vi "Dashboard Main.vi"() -> ()   [LabVIEW 2023]
uses:
  <vilib>/event_ctls.llb/eventvkey.ctl
  <vilib>/Rock Robotics/WPI/ThirdParty/JAS_Junk/TrajLib/TypeDef/TRANSLATION2D.ctl
  d5e2e769-f078-4149-bfe1-3f7844503895.vi
  <vilib>/Rock Robotics/WPI/ThirdParty/JAS_Junk/TrajLib/Conv_Radians_Deg.vi
  <vilib>/Rock Robotics/WPI/ThirdParty/JAS_Junk/TrajLib/Conv_Deg_Radians.vi
  <vilib>/Rock Robotics/WPI/ThirdParty/JAS_Junk/TrajLib/Translation2d_Create.vi
  <vilib>/Rock Robotics/WPI/ThirdParty/JAS_Junk/TrajLib/Rotation2d_CreateXY.vi
  <vilib>/Rock Robotics/WPI/ThirdParty/JAS_Junk/TrajLib/VI/Util_GetTime_U32.vi
  <vilib>/Rock Robotics/WPI/ThirdParty/JAS_Junk/TrajLib/Util_CalcDist.vi
  <vilib>/Rock Robotics/Network Tables/NT Read Numeric Array.vi
  <vilib>/Rock Robotics/WPI/ThirdParty/JAS_Junk/TrajLib/VI/Util_GetTime_U64.vi
  <vilib>/Rock Robotics/WPI/Dashboard/WPI_DashboardLogging Global.vi
  <vilib>/picture/picture.llb/Draw True-Color Pixmap.vi
  <vilib>/Rock Robotics/WPI/ThirdParty/JAS_Junk/TrajLib/Trajectory_Library.lvlib
  <vilib>/vision/NI_Vision_Development_Module.lvlib
  <vilib>/Utility/miscctls.llb/LVPointDoubleTypeDef.ctl
panel:
  in  "FF on?":bool=TRUE
  in  "Arm/ArmLength_Meters":dbl
  in  "Arm/Mass_Kg":dbl
  in  "PID gains":T1
  in  "FF params":T2={"Kg_Gravity_gain"=0.5, "phi_Equilibrium_phase_Deg"=0.0, "Ks"=0.03}
  in  "Arm/ArmAngle_Dmd_Deg":dbl
  out "ArmAngle_Deg":dbl
  out "ArmSpeed_RadPerSec":dbl
  in  "Camera Settings Right":T3={"Frame Rate"=30, "Compression"=30, "Size"=1, "DB Camera Config"=FALSE} {"Frame Rate" scale=1.0..30.0; "Compression" scale=100.0..-1.0; "Size" items=["640x480", "320x240", "160x120"]}
  in  "Camera Name Right":string(combo)="No Camera Selection"
  out "Camera Perf":string
  in  "Camera Settings":T3={"Frame Rate"=30, "Compression"=30, "Size"=1, "DB Camera Config"=FALSE} {"Frame Rate" scale=1.0..30.0; "Compression" scale=100.0..-1.0; "Size" items=["640x480", "320x240", "160x120"]}
  in  "TCP":refnum<k5>
  in  "Rec Mode":enum32{"Stop", "Record", "Playback"}(radio)
  out "Robot IP":string
  out "Image Message":string="Timeout in Camera Communications"
  in  "Dashboard Tab":T4(tab)
  in  "Select Auto":string(combo)="Select Autonomous ..."
  out "NT Connection":bool
  out "MotorChart R":cluster{"Numeric":dbl, "Numeric":dbl}(graph)
  out "MotorChart L":cluster{"Numeric":dbl, "Numeric":dbl}(graph)
  out "MotorSliders R":cluster{"MotorSlide1":dbl, "MotorSlide2":dbl} {"MotorSlide2" scale=-1.0..1.0 scale format="%#_2e"; "MotorSlide1" scale=-1.0..1.0 scale format="%#_2e"}
  out "MotorSliders L":cluster{"MotorSlide1":dbl, "MotorSlide2":dbl} {"MotorSlide2" scale=-1.0..1.0 scale format="%#_2e"; "MotorSlide1" scale=-1.0..1.0 scale format="%#_2e"}
  out "Gyro":dbl(knob) scale=0.0..360.0
  out "JS1 Z":dbl(slide) scale=-1.0..1.0 scale format="%#_2e"
  out "JS1 Graph":cluster{"X":dbl, "Y":dbl}[](graph)
  out "JS1 Buttons":T5
  out "JS2 Z":dbl(slide) scale=-1.0..1.0 scale format="%#_2e"
  out "JS2 Graph":cluster{"X":dbl, "Y":dbl}[](graph)
  out "JS2 Buttons":T5
  out "Mode":T6(ring)=enum."Auto Disabled"
  out "Right Camera Perf":cluster{"Bandwidth (Mbps)":dbl, "FPS":dbl}
  out "Camera Image Right":T7(plugin-control)
  in  "DB/String 9":string
  in  "DB/String 8":string
  in  "DB/String 7":string
  in  "DB/String 6":string
  in  "DB/String 5":string
  in  "DB/String 4":string
  in  "DB/String 3":string
  in  "DB/String 2":string
  in  "DB/String 1":string
  in  "DB/String 0":string
  in  "DB/Slider 0":dbl(slide) scale=0.0..5.0
  in  "DB/Slider 1":dbl(slide) scale=0.0..5.0
  in  "DB/Slider 2":dbl(slide) scale=0.0..5.0
  in  "DB/Slider 3":dbl(slide) scale=0.0..5.0
  out "DB/LED 3":bool
  out "DB/LED 2":bool
  out "DB/LED 1":bool
  out "DB/LED 0":bool
  in  "DB/Button 3":bool
  in  "DB/Button 2":bool
  in  "DB/Button 1":bool
  in  "DB/Button 0":bool caption="New Name"
  out "Arm Graph":cluster{dbl[], dbl[]}[](graph)
  out "time":dbl
  out "Field":cluster{dbl[], dbl[]}[](graph)
  out "Current Time":dbl
  in  "Test Slider":dbl(slide) scale=0.0..100.0 scale format="%#_3g"
  in  "On/Off":bool caption="Solenoid"
  in  "Test Name":u16(ring) items=["Select the test to run..."]
  in  "Test Tree":string(tree)
  in  "Motor":cluster{"Value":dbl, "Enable":bool} {"Value" scale=-1.0..1.0 scale format="%#_3g"}
  out "Progress":T8 {"Test Progress" scale=0.0..100.0}
  in  "Rev/Fwd":cluster{"Forward":bool, "Reverse":bool}
  in  "Test Ring":u16(ring) items=["Monochrome", "Color"]
  in  "CheckList":i32(listbox)
  out "Tree":string(tree)
  out "Camera Image":T7(plugin-control)
  out "Background":bool
  in  "Camera Name":string(combo)="No Camera Selection"
  # "Motor Type: Falcon 500"
  # "Gear Ratio: 11.652"
  # "HW"
  # "HW"
  # "Joysticks"
  # "Drive Motors"
  # "Front"
  # "Right"
  # "Left"
  # "Back"
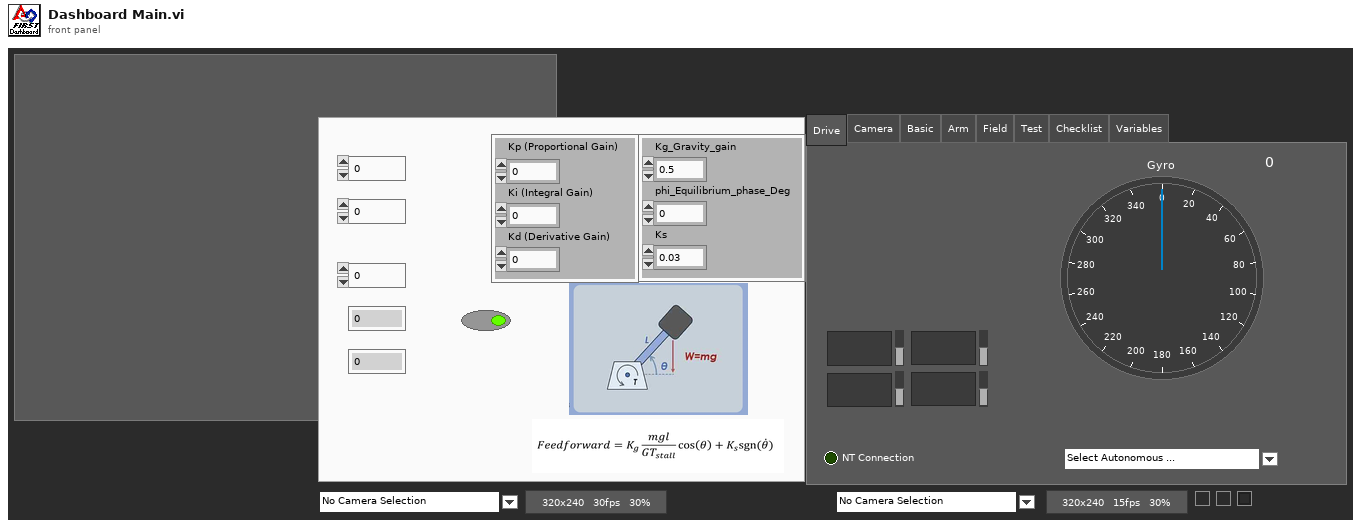
[diagram p1: front panel]
types:
  T1 = cluster{"Kp (Proportional Gain)":dbl, "Ki (Integral Gain)":dbl, "Kd (Derivative Gain)":dbl}
  T2 = cluster{"Kg_Gravity_gain":dbl, "phi_Equilibrium_phase_Deg":dbl, "Ks":dbl}
  T3 = cluster{"Frame Rate":i32, "Compression":i32, "Size":u16, "DB Camera Config":bool}
  T4 = enum32{"Drive", "Camera", "Basic", "Arm", "Field", "Test", "Checklist", "Variables"}
  T5 = cluster{bool, bool, bool, bool, bool, bool, bool, bool, bool, bool, bool, bool}
  T6 = enum8{"Tele-Op Disabled", "Tele-Op Enabled", "Auto Disabled", "Auto Enabled", "Test Disabled", "Test Enabled", "Disconnected", "No Code", "E-Stop"}
  T7 = typedef "IMAQ Image.ctl" = refnum<image>
  T8 = cluster{"Test Progress":u8, "Test Progress Text":string}
  T9 = typedef "Image Type" = u32
  T10 = cluster{"Save Path":path, "Interval (s)":dbl, "Keep":i32}
  T11 = enum32{"Drive", "Camera", "Basic", "Custom", "Test", "Commands", "Checklist", "Variables"}
  T12 = cluster{"Error Strings":string, "Disable Counts":cluster{u16, u16}, "Rail Faults":cluster{u16, u16, u16}, "Robot IP":string, "DB Mode":u8, "Event Info":cluster{"Name":string, "Type":u8, "Number":u16, "Replay":u8}}
  T13 = cluster{"Storage":cluster{"Disk Free":u64, "RAM Block":u32, "RAM free":u32}, "CPU Utilization":cluster{"CPU % ISR":sgl, "CPU % Time Crit":sgl, "CPU % Timed Str":sgl, "CPU % High":sgl, "CPU % Above":sgl, "CPU % Normal":sgl, "CPU % Low":sgl}, "CAN":cluster{"% Bus Utilization":sgl, "Bus Off Cnt":u32, "TX_FIFO Full Cnt":u32, "Receive Error Cnt":u8, "Transmit Error Cnt":u8}, "HID":cluster{"HID Outputs":u32, "Rumble Low":u16, "Rumble High":u16}[]}
  T14 = cluster{"Status bits":cluster{"Test Mode":bool, "Autonomous":bool, "Enabled":bool, "Code Start":bool, "Brownout":bool, "Reserved 2":bool, "Reserved 3":bool, "E-Stop":bool}, "Code Trace":cluster{"Disabled":bool, "TeleOp":bool, "Auto":bool, "Test":bool}, "Controller Type":enum16{"unknown", "cRIO", "roboRio"}, "Code?":enum16{"unknown", "noCode", "code"}, "Battery V":dbl}
  T15 = cluster{"Control Bits":cluster{"TestMode":bool, "Autonomous":bool, "Enabled":bool, "FMS Present":bool, bool, bool, bool, "E-Stop":bool}, "Team Station ":u8, "Countdown":sgl, "Joystick Values":cluster{"Axes":dbl[], "Buttons":bool[], "POVs":i16[]}[]}
  T16 = typedef "Trajectory_Library.lvlib/TRANSLATION2D.ctl" = cluster{"X":dbl, "Y":dbl}
  T17 = cluster{"Axes":dbl[], "Buttons":bool[], "POVs":i16[]}[]
  T18 = cluster{"Axes":dbl[], "Buttons":bool[], "POVs":i16[]}
  T19 = cluster{"Buttons[0]":bool, "Buttons[1]":bool, "Buttons[2]":bool, "Buttons[3]":bool, "Buttons[4]":bool, "Buttons[5]":bool, "Buttons[6]":bool, "Buttons[7]":bool, "Buttons[8]":bool, "Buttons[9]":bool, "Buttons[10]":bool, "Buttons[11]":bool}
  T20 = typedef "Trajectory_Library.lvlib/ROTATION2D.ctl" = cluster{"VALUE":dbl, "COS":dbl, "SIN":dbl}
  T21 = cluster{"Camera Image":refnum<vi>, "Dashboard Tab":refnum<vi>, "Background":refnum<vi>, "Rec Mode":refnum<vi>, "Test Slider":refnum<vi>, "On/Off ":refnum<vi>, "Test Ring":refnum<vi>, "Rev/Fwd":refnum<vi>, "Test Name":refnum<vi>, "Motor":refnum<vi>, "Progress":refnum<vi>, "CheckList":refnum<vi>, "Tree":refnum<vi>, "Test Tree":refnum<vi>, "Camera Settings":refnum<vi>, "Camera Name":refnum<vi>, "Camera Perf":refnum<vi>, "Camera Settings Right":refnum<vi>, "Camera Name Right":refnum<vi>, "Camera Image Right":refnum<vi>}
  T22 = cluster{"Global Rectangle":i32[], "Contours":cluster{"Contour Type":u32, "ROI Type":u32, "Points":i32[]}[]}
  T23 = cluster{"Camera Name":string, string, "Saved DB Images Info":cluster{"Save Path":path, "Interval (s)":dbl, "Keep":i32}}
  T24 = cluster{"Camera Name Right":string, string, "Saved DB Images Info":cluster{"Save Path":path, "Interval (s)":dbl, "Keep":i32}}
  T25 = cluster{"Operation":enum16{"Update", "Clear"}, "Color Box":u32}[]
  T26 = typedef "eventvkey.ctl" = enum16{"ASCII", "Enter", "Return", "Shift", "Ctrl", "Alt", "Cmd", "Opt", "Caps", "NumLock", "Clear", "Break", "Up", "Down", "Left", "Right", "Insert", "Delete", "Home", "End", "PageUp", "PageDown", "Escape", "Help", "Pause", "ScrollLock", "F1", "F2", "F3", "F4", "F5", "F6", "F7", "F8", "F9", "F10", "F11", "F12", "F13", "F14", "F15", "F16", "F17", "F18", "F19", "F20", "F21", "F22", "F23", "F24", "Play", "VolumeUp", "VolumeDown", "Mute", "Two Byte Char"}
  T27 = cluster{"Image Size":bool, "Image Type":bool, "Pixel Value":bool, "ROI Information":bool, "Zoom Factor":bool}
  T28 = cluster{"Operation":enum16{"Update", "Clear"}, "Color Box":u32}
  T29 = cluster{"Shift":bool, "Ctrl":bool, "Alt":bool, "Cmd":bool, "Opt":bool}
  T30 = typedef "imagedata.ctl" = cluster{"image type":i32, "image depth":i32, "image":u8[], "mask":u8[], "colors":u32[], "Rectangle":cluster{"left":i16, "top":i16, "right":i16, "bottom":i16}}
  T31 = typedef "LVPointDoubleTypeDef.ctl" = cluster{"X":dbl, "Y":dbl}
  T32 = typedef "LVCursorListTypeDef.ctl" = cluster{"Name":string, "Color":u32, "Style":u8, "Point Style":u8, "Name Visible":bool, "Allow Drag":bool, "Cursor Mode":u32, "Plot":i32, "Index":i32, "Position":cluster{"X":dbl, "Y":dbl}, "X Scale":u32, "Y Scale":u32, "Watch Plots":i32[], "Watch All Plots":bool, "Plot Area":i32, "Label Offset":cluster{"X":dbl, "Y":dbl}}[]
  T33 = cluster{"Name":string, "Color":u32, "Style":u8, "Point Style":u8, "Name Visible":bool, "Allow Drag":bool, "Cursor Mode":u32, "Plot":i32, "Index":i32, "Position":cluster{"X":dbl, "Y":dbl}, "X Scale":u32, "Y Scale":u32, "Watch Plots":i32[], "Watch All Plots":bool, "Plot Area":i32, "Label Offset":cluster{"X":dbl, "Y":dbl}}
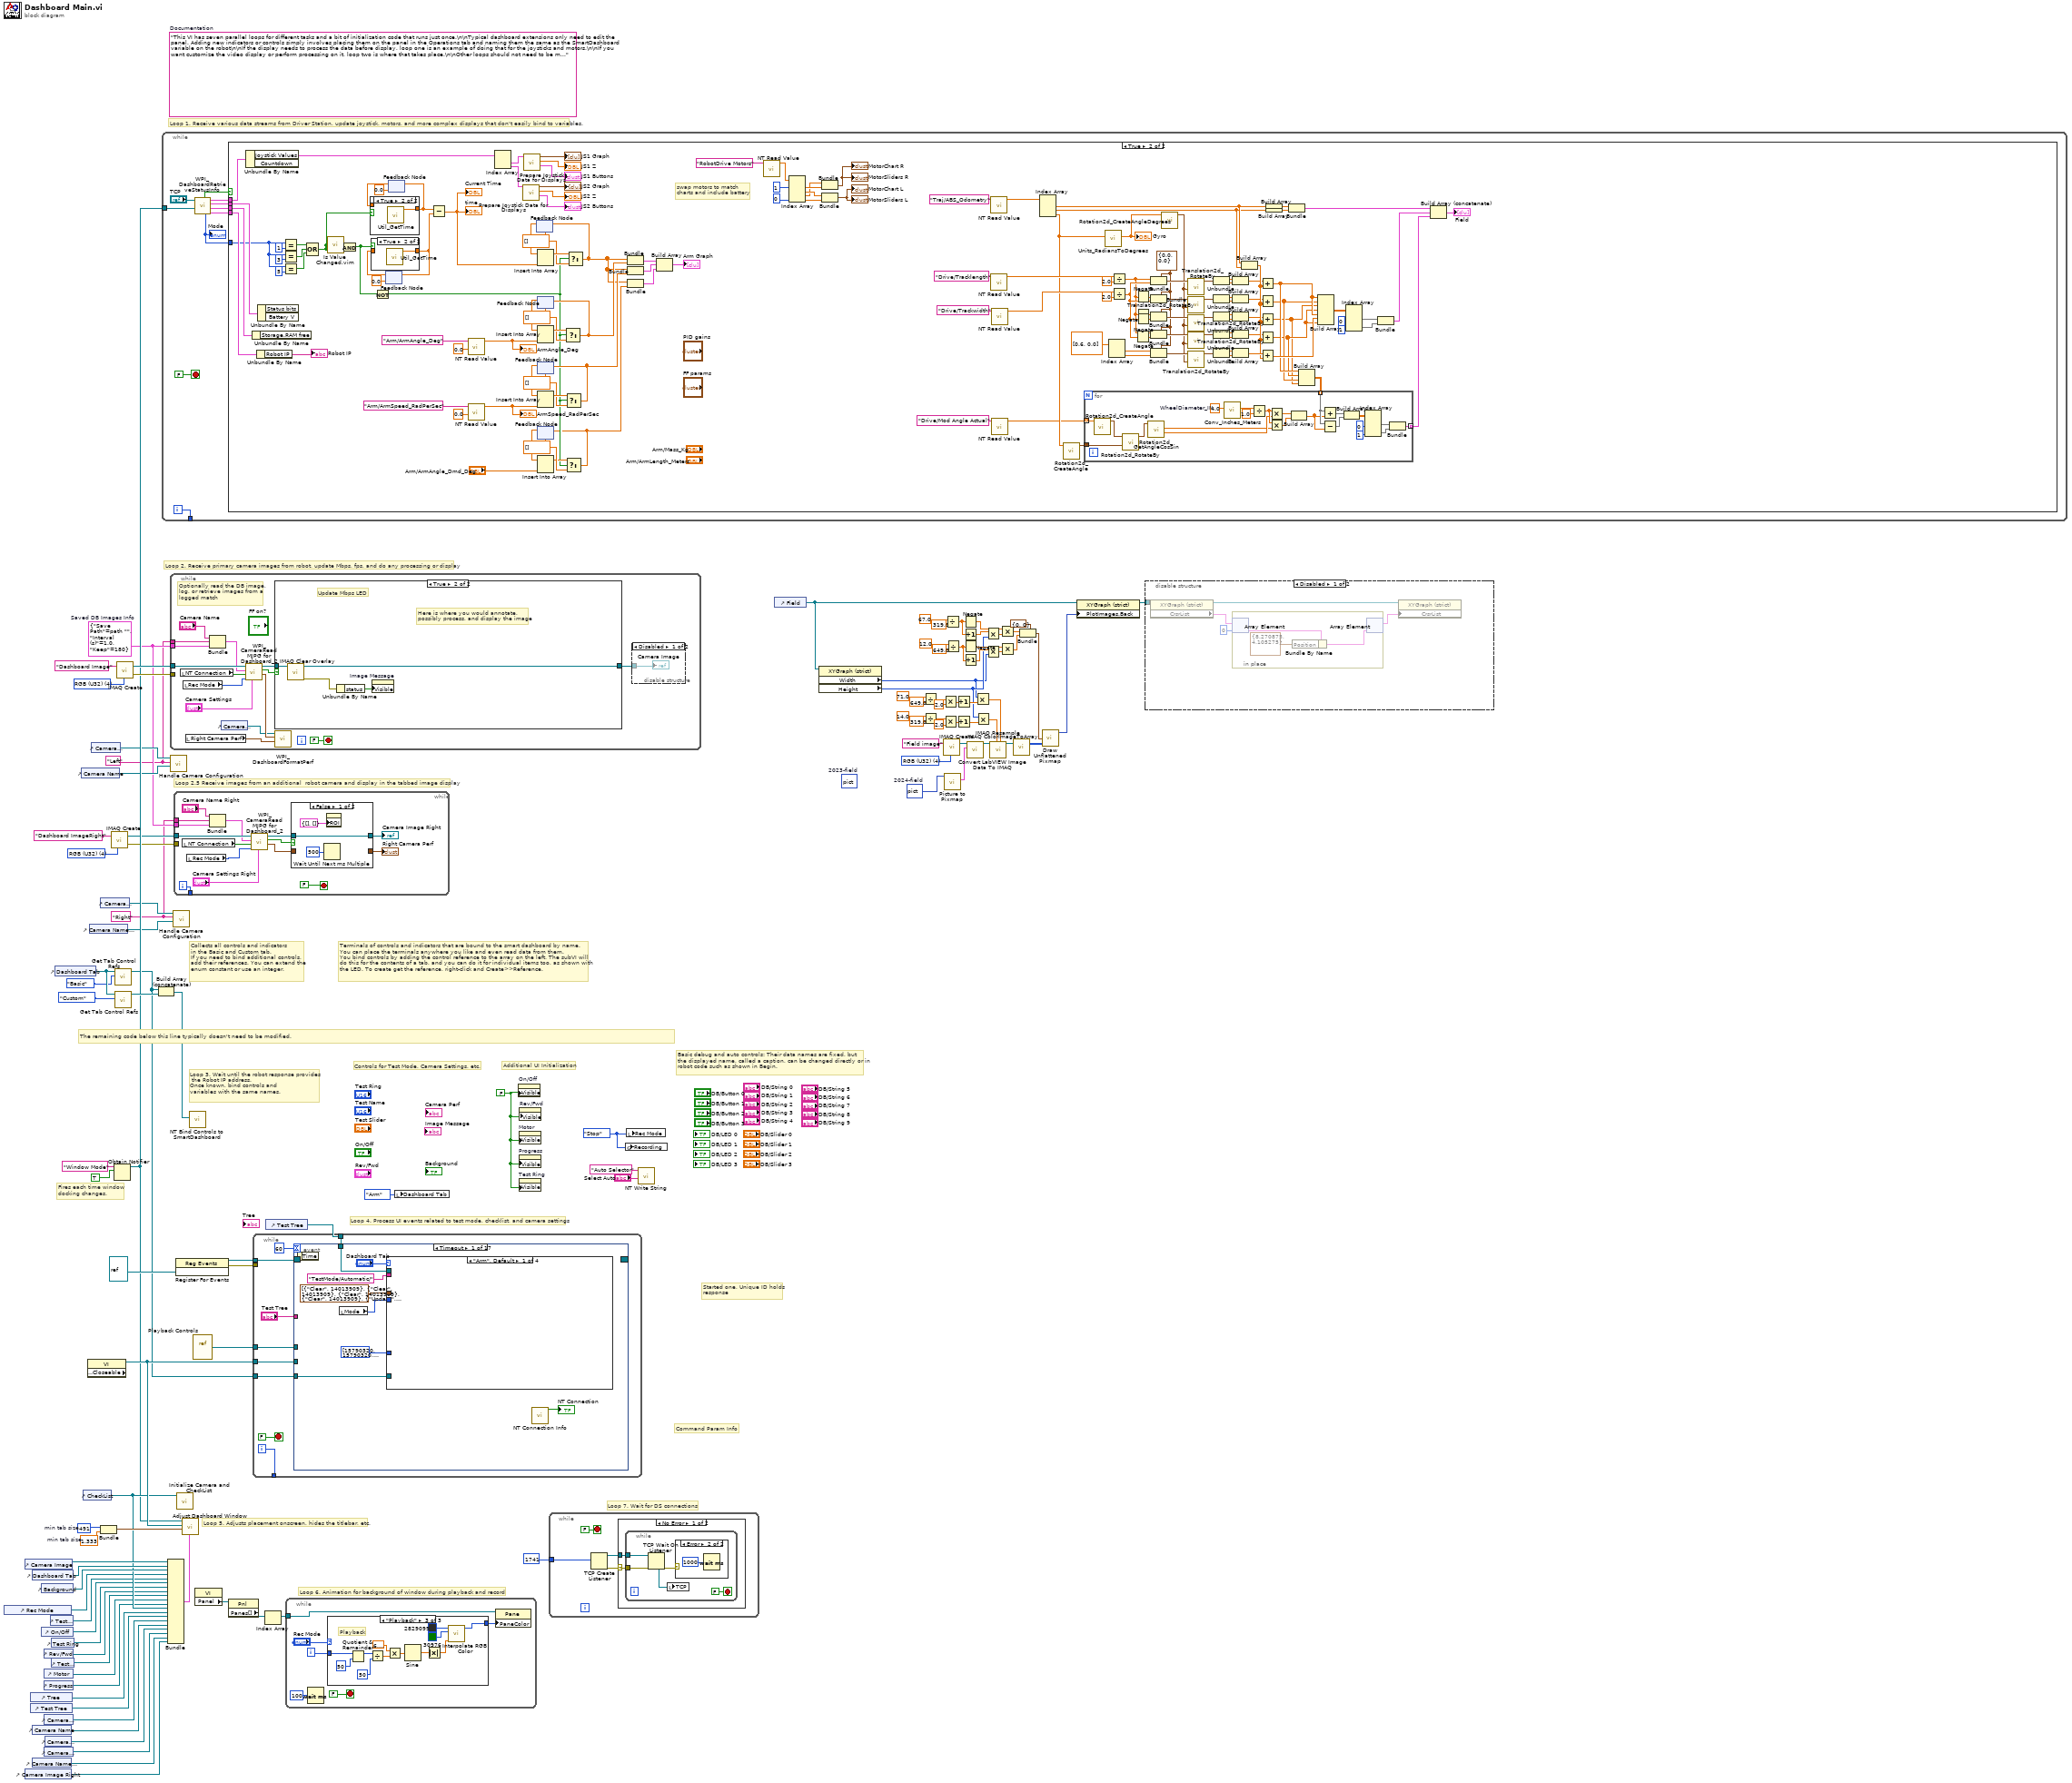
[diagram p0: block diagram]
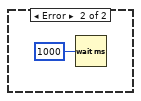
[diagram p5: hidden frame]
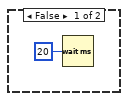
[diagram p6: hidden frame]
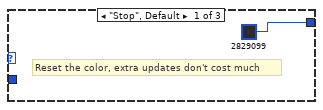
[diagram p9: hidden frame]
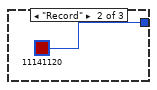
[diagram p10: hidden frame]
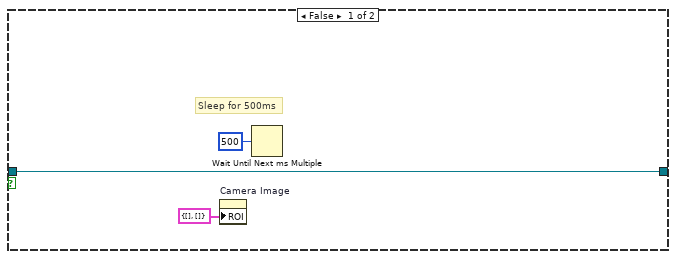
[diagram p12: hidden frame]
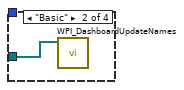
[diagram p13: hidden frame]
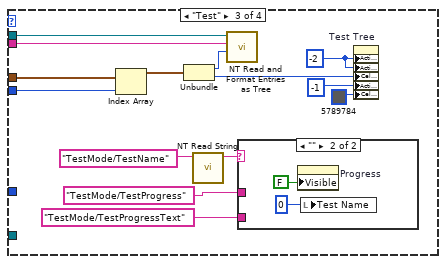
[diagram p14: hidden frame]
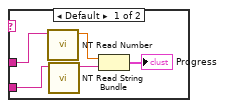
[diagram p15: hidden frame]
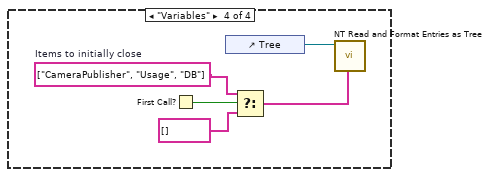
[diagram p16: hidden frame]
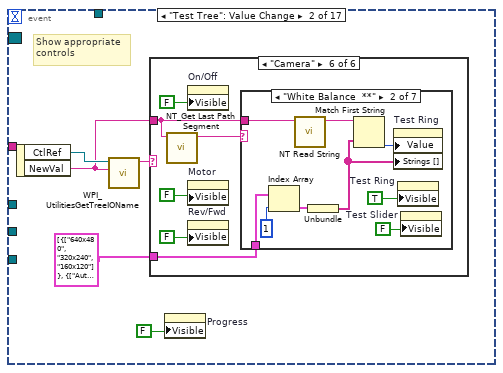
[diagram p17: hidden frame]
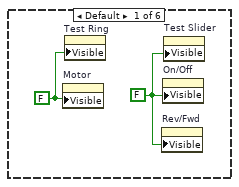
[diagram p18: hidden frame]
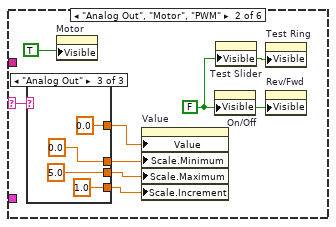
[diagram p19: hidden frame]
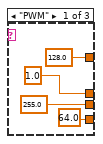
[diagram p20: hidden frame]
diagram:
  w3 = picture bytes[2013030]  # 2024-field
  w43 = T9 4 items=["Grayscale (U8)", "Grayscale (I16)", "Grayscale (SGL)", "Complex (CSG)", "RGB (U32)", "HSL (U32)", "RGB (U64)", "Grayscale (U16)"] ("Image Type")
  (unwired) picture bytes[1973190]  # 2023-field
  w47 = T10 {"Save Path"=path "", "Interval (s)"=1.0, "Keep"=180}  # Saved DB Images Info
  w46 = "Right"
  w45 = "Left"
  w57 = T9 4 items=["Grayscale (U8)", "Grayscale (I16)", "Grayscale (SGL)", "Complex (CSG)", "RGB (U32)", "HSL (U32)", "RGB (U64)"] ("Image Type")
  w85 = 491  # min tab size
  w84 = 1.333  # min tab size
  w92 = enum32{"Stop", "Record", "Playback"}."Stop" ("Rec Mode")
  w69 = FALSE ("Visible")
  (unwired) "This VI has seven parallel loops for different tasks and a bit of initialization code that runs just once.\n\nTypical dashboard extensions only need to edit the panel. Adding new indicators or controls simply involves placing them on the panel in the Operations tab and naming them the same as the SmartDashboard variable on the robot\n\nIf the display needs to process the data before display, loop one is an example of doing that for the joysticks and motors.\n\nIf you want customize the video display or perform processing on it, loop two is where that takes place.\n\nOther loops should not need to be modified. They are pretty standard, and document the task they perform."  # Documentation
  w106 = T9 4 items=["Grayscale (U8)", "Grayscale (I16)", "Grayscale (SGL)", "Complex (CSG)", "RGB (U32)", "HSL (U32)", "RGB (U64)"] ("Image Type")
  # "Loop 2.5 Receive images from an additional  robot camera and display in the tabbed image display"
  # "Command Param Info"
  # "Started one, Unique ID holds\nresponse"
  # "Loop 7. Wait for DS connections"
  # "Basic debug and auto controls: Their data names are fixed, but\nthe displayed name, called a caption, can be changed directly or in\nrobot code such as shown in Begin."
  # "Controls for Test Mode, Camera Settings, etc."
  # "Additional UI Initialization"
  # "Loop 6. Animation for background of window during playback and record"
  # "Fires each time window\ndocking changes."
  # "Collects all controls and indicators\nin the Basic and Custom tab.\nIf you need to bind additional controls,\nadd their references. You can extend the\nenum constant or use an integer."
  # "The remaining code below this line typically doesn't need to be modified."
  # "Loop 4. Process UI events related to test mode, checklist, and camera settings"
  # "Terminals of controls and indicators that are bound to the smart dashboard by name.\nYou can place the terminals anywhere you like and even read data from them.\nYou bind controls by adding the control reference to the array on the left. The subVI will\ndo this for the contents of a tab, and you can do it for individual items too, as shown with\nthe LED. To create get the reference, right-click and Create>>Reference."
  # "Loop 3. Wait until the robot response provides\n the Robot IP address.\nOnce known, bind controls and\nvariables with the same names."
  # "Loop 5. Adjusts placement onscreen, hides the titlebar, etc."
  # "Loop 1. Receive various data streams from Driver Station, update joystick, motors, and more complex displays that don't easily bind to variables."
  # "Loop 2. Receive primary camera images from robot, update Mbps, fps, and do any processing or display"
  n1 = control-ref of="Rec Mode"() -> (w75:refnum<vi>)
  n2 = control-ref of="Camera Image Right"() -> (w50:refnum<vi>)
  n3 = control-ref of="Camera Image"() -> (w87:refnum<vi>)
  n4 = control-ref of="Tree"() -> (w79:refnum<vi>)
  n5 = control-ref of="Test Tree"() -> (w78:refnum<vi>)
  n6 = control-ref of="Dashboard Tab"() -> (w86:refnum<vi>)
  n7 = control-ref of="Camera Name"() -> (w63:refnum<vi>)
  n8 = control-ref of="Camera Name Right"() -> (w51:refnum<vi>)
  n9 = control-ref of="Background"() -> (w82:refnum<vi>)
  n10 = control-ref of="On/Off"() -> (w73:refnum<vi>)
  n11 = control-ref of="Progress"() -> (w70:refnum<vi>)
  n12 = control-ref of="Camera Settings"() -> (w64:refnum<vi>)
  n13 = control-ref of="Camera Settings Right"() -> (w52:refnum<vi>)
  n14 = control-ref of="Rev/Fwd"() -> (w71:refnum<vi>)
  n15 = control-ref of="Motor"() -> (w76:refnum<vi>)
  n16 = control-ref of="Camera Perf"() -> (w62:refnum<vi>)
  n17 = control-ref of="Test Slider"() -> (w74:refnum<vi>)
  n18 = control-ref of="Test Ring"() -> (w72:refnum<vi>)
  n19 = control-ref of="Test Name"() -> (w77:refnum<vi>)
  n20 = control-ref of="Dashboard Tab"() -> (w90:refnum<vi>)
  n21 = control-ref of="Camera Name"() -> (w65:refnum<vi>)
  n22 = control-ref of="CheckList"() -> (w80:refnum<vi>)
  n23 = property class="VI" props=["Front Panel.Closeable"]() -> (reference out=w91:refnum<vi>)  [unwired: 2 in, 2 out]
  n24 = control-ref of="Camera Name Right"() -> (w53:refnum<vi>)
  n25 = control-ref of="Camera Settings"() -> (w66:refnum<vi>)
  n26 = control-ref of="Camera Settings Right"() -> (w54:refnum<vi>)
  n27 = Bundle("min tab size"=w85, "min tab size"=w84) -> (w83:cluster{"min tab size":i32, "min tab size":dbl})  [unwired: 1 in]
  n28 = call "IMAQ Create"("Image Name"="Dashboard ImageRight", "Image Type"=w57) -> ("New Image"=w56:T7, "error out"=w55:errorcluster)  [unwired: 2 in, 1 out]
  n29 = Obtain Notifier(name (unnamed)="Window Mode", notification data type=TRUE) -> (notifier out=w68:refnum<notifier>)  [unwired: 2 in, 2 out]
  n30 = call <vilib>:"Get Tab Control Refs.vi"("Page Index"=T11."Basic" ("Dashboard Tab"), "TabControl in"=w90) -> ("ControlsOnPage"=w61:refnum<vi>[])  [unwired: 9 in]
  n31 = call <vilib>:"Get Tab Control Refs.vi"("Page Index"=T11."Custom" ("Dashboard Tab"), "TabControl in"=w90) -> ("ControlsOnPage"=w89:refnum<vi>[])  [unwired: 9 in]
  n32 = call "IMAQ Create"("Image Name"="Dashboard Image", "Image Type"=w106) -> ("New Image"=w104:T7, "error out"=w103:errorcluster)  [unwired: 2 in, 1 out]
  n33 = Build Array (concatenate)(w61, w89) -> (w88:refnum<vi>[])
  n34 = while {
    tunnel: [w115] -> _
    tunnel: w68 -> [w107]
    i -> [w115]
    stop <- FALSE stop-if-true
    n35 = call <vilib>:"WPI_DashboardRetrieveStatusInfo.vi"("Window Mode Notifier"=w107, "TCP Cnx"="TCP") -> ("Power and Errors"=w110:T12, "Robot Metrics"=w113:T13, "Status Info"=w114:T14, "Control Info"=w111:T15, "Robot Mode"=w109:T6, "Process?"=w112:bool)  [unwired: 4 in]
    "Mode" <- w109
    n36 = case shown="True" w112 {
      tunnel: w114 -> [_ w255]
      tunnel: w113 -> [_ w254]
      tunnel: w111 -> [_ w253]
      tunnel: w110 -> [_ w252]
      tunnel: w109 -> [_ w152]
      frame False {
        n37 = Wait (ms)(milliseconds to wait=u32 20) -> ()  [unwired: 1 out]
      }
      frame True {
        w123 = dbl[] []
        w147 = dbl[] []
        w174 = T16 {"X"=0.0, "Y"=0.0} ("In Translation")
        w146 = dbl[] []
        w145 = dbl[] []
        # "swap motors to match\ncharts and include battery"
        n38 = Unbundle By Name(w253) -> ("Joystick Values"=w243:T17)  [unwired: 1 out]
        n39 = Unbundle By Name(w254) -> ()  [unwired: 1 out]
        n40 = Unbundle By Name(w252) -> ("Robot IP"=→"Robot IP":string)
        n41 = Unbundle By Name(w255) -> ()  [unwired: 2 out]
        n42 = Equal?(x=w152, y=u32 1) -> (x = y?=w151:bool)
        n43 = Equal?(x=w152, y=u32 3) -> (x = y?=w150:bool)
        n44 = Equal?(x=w152, y=u32 5) -> (x = y?=w149:bool)
        n45 = Compound Arithmetic op=OR(w151, w150, w149) -> (w148:bool)
        n46 = call "Is Value Changed.vim"("value"=w148) -> ("changed or first call?"=w226:bool)
        n47 = And(x=w226, y=w148) -> (x .and. y?=w216:bool)
        n48 = Not(x=w216) -> (.not. x?=w120:bool)
        n49 = feedback #1(0.0 ("FPGA_Time_Seconds")) -> (w230:dbl)
        n50 = case shown="True" w216 {
          tunnel: [w280 w281] -> w229
          tunnel: w230 -> [w280 _]
          frame False {
          }
          frame True {
            n51 = call <vilib>:"Util_GetTime.vi"() -> ("FPGA_Time_Seconds"=w281:dbl)  [unwired: 9 in, 2 out]
          }
        }
        n52 = feedback-in #1(w229) -> ()
        n53 = feedback #2(0.0 ("FPGA_Time_Seconds")) -> (w221:dbl)
        n54 = case shown="True" w148 {
          tunnel: [w278 w279] -> w220
          tunnel: w221 -> [w278 _]
          frame False {
          }
          frame True {
            n55 = call <vilib>:"Util_GetTime.vi"() -> ("FPGA_Time_Seconds"=w279:dbl)  [unwired: 9 in, 2 out]
          }
        }
        n56 = feedback-in #2(w220) -> ()
        n57 = Subtract(x=w220, y=w229) -> (x-y=w214:dbl)
        "time" <- w214
        "Current Time" <- w214
        n58 = call-poly <vilib>:"NT Read Value.vi"("default value"=0.0, "name"="Arm/ArmAngle_Deg" ("PV (NT Name)")) -> ("value"=w223:dbl)  [unwired: 7 in, 2 out]
        "ArmAngle_Deg" <- w223
        n59 = call-poly <vilib>:"NT Read Value.vi"("default value"=0.0, "name"="Arm/ArmSpeed_RadPerSec" ("ArmVelocity (NT Name)")) -> ("value"=w157:dbl)  [unwired: 7 in, 2 out]
        "ArmSpeed_RadPerSec" <- w157
        n60 = Index Array(array=w243) -> (element #1=w242:T18, element #2=w238:T18)  [unwired: 2 in]
        n61 = call "Prepare Joystick Data for Displays.vi"("Joystick Values"=w238) -> ("Buttons"=→"JS2 Buttons":T19, "Z Axis"=→"JS2 Z":dbl, "Cartesian Data"=→"JS2 Graph":cluster{"X axis":dbl, "X axis":dbl}[])  [unwired: 8 in]
        n62 = call "Prepare Joystick Data for Displays.vi"("Joystick Values"=w242) -> ("Buttons"=→"JS1 Buttons":T19, "Z Axis"=→"JS1 Z":dbl, "Cartesian Data"=→"JS1 Graph":cluster{"X axis":dbl, "X axis":dbl}[])  [unwired: 8 in]
        n63 = feedback #3(w145) -> (w225:dbl[])
        n64 = Insert Into Array(array=w225, new element=w214) -> (w218:dbl[])  [unwired: 1 in]
        n65 = feedback #4(w146) -> (w224:dbl[])
        n66 = Insert Into Array(array=w224, new element=w223) -> (w217:dbl[])  [unwired: 1 in]
        n67 = feedback #5(w147) -> (w158:dbl[])
        n68 = Insert Into Array(array=w158, new element=w157) -> (w156:dbl[])  [unwired: 1 in]
        n69 = feedback #6(w123) -> (w121:dbl[])
        n70 = Insert Into Array(array=w121, new element="Arm/ArmAngle_Dmd_Deg") -> (w122:dbl[])  [unwired: 1 in]
        n71 = Select(t=w217, s=w120, f=w146) -> (s? t:f=w144:dbl[])
        n72 = feedback-in #4(w144) -> ()
        n73 = Select(t=w156, s=w120, f=w147) -> (s? t:f=w155:dbl[])
        n74 = feedback-in #5(w155) -> ()
        n75 = Select(t=w122, s=w120, f=w123) -> (s? t:f=w119:dbl[])
        n76 = feedback-in #6(w119) -> ()
        n77 = Select(t=w218, s=w120, f=w145) -> (s? t:f=w124:dbl[])
        n78 = feedback-in #3(w124) -> ()
        n79 = Bundle(w124, w144) -> (w222:cluster{dbl[], dbl[]})  [unwired: 1 in]
        n80 = Bundle(w124, w155) -> (w126:cluster{dbl[], dbl[]})  [unwired: 1 in]
        n81 = Bundle(w124, w119) -> (w125:cluster{dbl[], dbl[]})  [unwired: 1 in]
        n82 = Build Array(w222, w126, w125) -> (→"Arm Graph":cluster{dbl[], dbl[]}[])
        n83 = call-poly <vilib>:"NT Read Value.vi"("name"="RobotDrive Motors" ("Name")) -> ("value"=w233:dbl[])  [unwired: 8 in, 2 out]
        n84 = Index Array(array=w233, index #1=1, index #4=0) -> (element #1=w247:dbl, element #2=w248:dbl, element #3=w246:dbl, element #4=w251:dbl)  [unwired: 2 in]
        n85 = Bundle("Numeric"=w246, "Numeric"=w247) -> (→"MotorChart R" →"MotorSliders R":cluster{"Numeric":dbl, "Numeric":dbl})  [unwired: 1 in]
        n86 = Bundle("Numeric"=w248, "Numeric"=w251) -> (→"MotorChart L" →"MotorSliders L":cluster{"Numeric":dbl, "Numeric":dbl})  [unwired: 1 in]
        n87 = call-poly <vilib>:"NT Read Value.vi"("name"="Traj/ABS_Odometry") -> ("value"=w172:dbl[])  [unwired: 8 in, 2 out]
        n88 = call-poly <vilib>:"NT Read Value.vi"("name"="Drive/Tracklength" ("Name")) -> ("value"=w162:dbl)  [unwired: 8 in, 2 out]
        n89 = call-poly <vilib>:"NT Read Value.vi"("name"="Drive/Trackwidth" ("Name")) -> ("value"=w161:dbl)  [unwired: 8 in, 2 out]
        n90 = call-poly <vilib>:"NT Read Value.vi"("name"="Drive/Mod Angle Actual") -> ("value"=w128:dbl[])  [unwired: 8 in, 2 out]
        n91 = Index Array(array=w172) -> (element #1=w171:dbl, element #2=w170:dbl, element #3=w133:dbl)  [unwired: 3 in]
        n92 = call <vilib>:"Rotation2d_CreateAngle.vi"("Angle"=w133) -> ("ROTATION"=w130:T20)  [unwired: 10 in]
        n93 = call <vilib>:"Units_RadiansToDegrees.vi"("Radians"=w133) -> ("Degrees"=w160:dbl)  [unwired: 10 in]
        "Gyro" <- w160
        n94 = Index Array(array=dbl[] [0.6, 0.0] ("y")) -> (element #1=w176:dbl, element #2=w175:dbl)  [unwired: 2 in]
        n95 = Divide(x=w162, y=2.0) -> (x/y=w199:dbl)
        n96 = Divide(x=w161, y=2.0) -> (x/y=w200:dbl)
        n97 = Negate(x=w200) -> (-x=w182:dbl)
        n98 = Negate(x=w199) -> (-x=w203:dbl)
        n99 = Negate(x=w199) -> (-x=w202:dbl)
        n100 = Negate(x=w200) -> (-x=w201:dbl)
        n101 = Bundle(cluster=w174, "X"=w199, "Y"=w200) -> (w211:T16)
        n102 = Bundle(cluster=w174, "X"=w203, "Y"=w200) -> (w207:T16)
        n103 = Bundle(cluster=w174, "X"=w202, "Y"=w201) -> (w206:T16)
        n104 = Bundle(cluster=w174, "X"=w199, "Y"=w182) -> (w205:T16)
        n105 = Bundle(cluster=w174, "X"=w176, "Y"=w175) -> (w183:T16)
        n106 = call <vilib>:"Rotation2d_CreateAngleDegrees.vi"("Angle_Degrees"=w160) -> ("ROTATION"=w181:T20)  [unwired: 10 in]
        n107 = call <vilib>:"Translation2d_RotateBy.vi"("other Rotation"=w181, "In Translation"=w211) -> ("Out Translation"=w210:T16)  [unwired: 9 in]
        n108 = call <vilib>:"Translation2d_RotateBy.vi"("other Rotation"=w181, "In Translation"=w207) -> ("Out Translation"=w209:T16)  [unwired: 9 in]
        n109 = call <vilib>:"Translation2d_RotateBy.vi"("other Rotation"=w181, "In Translation"=w206) -> ("Out Translation"=w208:T16)  [unwired: 9 in]
        n110 = call <vilib>:"Translation2d_RotateBy.vi"("other Rotation"=w181, "In Translation"=w205) -> ("Out Translation"=w204:T16)  [unwired: 9 in]
        n111 = call <vilib>:"Translation2d_RotateBy.vi"("other Rotation"=w181, "In Translation"=w183) -> ("Out Translation"=w184:T16)  [unwired: 9 in]
        n112 = Unbundle(w210) -> ("X"=w198:dbl, "Y"=w197:dbl)
        n113 = Unbundle(w209) -> ("X"=w195:dbl, "Y"=w196:dbl)
        n114 = Unbundle(w208) -> ("X"=w194:dbl, "Y"=w193:dbl)
        n115 = Unbundle(w204) -> ("X"=w192:dbl, "Y"=w191:dbl)
        n116 = Unbundle(w184) -> ("X"=w180:dbl, "Y"=w185:dbl)
        n117 = Build Array(w198, w197) -> (w141:dbl[])
        n118 = Build Array(w195, w196) -> (w140:dbl[])
        n119 = Build Array(w194, w193) -> (w138:dbl[])
        n120 = Build Array(w192, w191) -> (w139:dbl[])
        n121 = Build Array(w180, w185) -> (w179:dbl[])
        n122 = Build Array(w171, w170) -> (w173:dbl[])
        n123 = Add(x=w141, y=w173) -> (x+y=w137:dbl[])
        n124 = Add(x=w140, y=w173) -> (x+y=w136:dbl[])
        n125 = Add(x=w138, y=w173) -> (x+y=w134:dbl[])
        n126 = Add(x=w139, y=w173) -> (x+y=w135:dbl[])
        n127 = Add(x=w179, y=w173) -> (x+y=w178:dbl[])
        n128 = Build Array(w171) -> (w169:dbl[])
        n129 = Build Array(w170) -> (w168:dbl[])
        n130 = Bundle(w169, w168) -> (w167:cluster{dbl[], dbl[]})  [unwired: 1 in]
        n131 = Build Array(w137, w135, w136, w134) -> (w131:dbl[][])
        n132 = for {
          tunnel: w131 -> [w274] mode=indexing
          tunnel: [w264] -> w129 mode=indexing
          tunnel: w130 -> [w259]
          tunnel: w128 -> [w257] mode=indexing
          w258 = 4.0  # WheelDiameter_IN
          n133 = call <vilib>:"Rotation2d_CreateAngle.vi"("Angle"=w257) -> ("ROTATION"=w256:T20)  [unwired: 10 in]
          n134 = call <vilib>:"Rotation2d_RotateBy.vi"("other Rotation"=w259, "in ROTATION"=w256) -> ("out ROTATION"=w260:T20)  [unwired: 9 in]
          n135 = call <vilib>:"Rotation2d_GetAngleCosSin.vi"("in ROTATION"=w260) -> ("Cosine"=w273:dbl, "Sine"=w272:dbl)  [unwired: 8 in, 1 out]
          n136 = call <vilib>:"Conv_Inches_Meters.vi"("INCH"=w258) -> ("Meters"=w276:dbl)  [unwired: 10 in]
          n137 = Divide(x=w276, y=1.0) -> (x/y=w275:dbl)
          n138 = Multiply(x=w275, y=w273) -> (x*y=w262:dbl)
          n139 = Multiply(x=w275, y=w272) -> (x*y=w263:dbl)
          n140 = Build Array(w262, w263) -> (w261:dbl[])
          n141 = Add(x=w274, y=w261) -> (x+y=w271:dbl[])
          n142 = Subtract(x=w274, y=w261) -> (x-y=w270:dbl[])
          n143 = Build Array(w271, w270) -> (w267:dbl[][])
          n144 = Index Array(array=w267, index (col) #1=0 ("disabled index (col)"), index (col) #2=1 ("index (col)")) -> (element #1=w265:dbl[], element #2=w266:dbl[])  [unwired: 2 in]
          n145 = Bundle(w265, w266) -> (w264:cluster{dbl[], dbl[]})  [unwired: 1 in]
        }
        n146 = Build Array(w137, w136, w134, w135, w137, w178, w135) -> (w190:dbl[][])
        n147 = Index Array(array=w190, index (col) #1=0 ("disabled index (col)"), index (col) #2=1 ("index (col)")) -> (element #1=w188:dbl[], element #2=w186:dbl[])  [unwired: 2 in]
        n148 = Bundle(w188, w186) -> (w166:cluster{dbl[], dbl[]})  [unwired: 1 in]
        n149 = Build Array (concatenate)(w167, w166, w129) -> (→"Field":cluster{dbl[], dbl[]}[])
      }
    }
  }
  n150 = Bundle("Camera Image"=w87, "Dashboard Tab"=w86, "Background"=w82, "Rec Mode"=w75, "Test Slider"=w74, "On/Off"=w73, "Test Ring"=w72, "Rev/Fwd"=w71, "Test Name"=w77, "Motor"=w76, "Progress"=w70, "CheckList"=w80, "Tree"=w79, "Test Tree"=w78, "Camera Settings"=w64, "Camera Name"=w63, "Camera Perf"=w62, "Camera Settings Right"=w52, "Camera Name Right"=w51, "Camera Image Right"=w50) -> (w81:T21)  [unwired: 1 in]
  n151 = call "Handle Camera Configuration.vi"("CameraNameRef"=w65, "Display Name"=w45, "ClusterRef"=w66) -> ()  [unwired: 9 in]
  n152 = while {
    tunnel: w104 -> [w295]
    tunnel: w103 -> [_]
    tunnel: w47 -> [w288]
    tunnel: w45 -> [w285]
    stop <- FALSE stop-if-true
    # "Optionally read the DB image,\nlog, or retrieve images from a\nlogged match"
    n153 = local read "NT Connection"() -> (w289:bool)
    n154 = local read "Rec Mode"() -> (w292:enum32{"Stop", "Record", "Playback"})
    n155 = local read "Right Camera Perf"() -> (w283:cluster{"Bandwidth (Mbps)":dbl, "FPS":dbl})
    n156 = Bundle("Camera Name"="Camera Name", w285, "Saved DB Images Info"=w288) -> (w287:T23)  [unwired: 1 in]
    n157 = control-ref of="Camera Perf"() -> (w282:refnum<vi>)
    n158 = call <vilib>:"WPI_CameraRead MJPG for Dashboard_2.vi"("Camera Settings"="Camera Settings", "Rec Mode"=w292, "NT Connection"=w289, "Capture Info"=w287, "Image in"=w295) -> ("perf info"=w284:cluster{"Bandwidth (Mbps)":dbl, "fps":dbl}, "Active"=w293:bool, "Image\\ out"=w294:T7)  [unwired: 4 in]
    n159 = case shown="True" w293 {
      tunnel: w294 -> [w299 w302]
      tunnel: [w299 w301] -> w290
      frame False {
        # "Sleep for 500ms"
        n160 = property on="Camera Image" class="ImageControl"("ROI"=T22 {"Global Rectangle"=[], "Contours"=[]}) -> ()  [unwired: 2 in, 2 out]
        n161 = Wait Until Next ms Multiple(millisecond multiple=u32 500) -> ()  [unwired: 1 out]
      }
      frame True {
        # "Here is where you would annotate,\npossibly process, and display the image"
        # "Update Mbps LED"
        n162 = call "IMAQ Clear Overlay"("Image"=w302) -> ("error out"=w303:errorcluster, "Image Out"=w301:T7)  [unwired: 2 in, 7 out]
        n163 = Unbundle By Name(w303) -> ("status"=w304:bool)
        n164 = property on="Image Message" class="Str"("Visible"=w304) -> ()  [unwired: 2 in, 2 out]
      }
    }
    n165 = call <vilib>:"WPI_DashboardFormatPerf.vi"("Right Camera Perf"=w283, "Performance"=w284, "String in"=w282) -> ()  [unwired: 9 in]
    n166 = disable-structure shown="Disabled" {
      disable-tunnel: w290 -> [w297 _]
      frame Disabled {
        "Camera Image" <- w297
      }
      frame Enabled {
      }
    }
  }
  n167 = call "Handle Camera Configuration.vi"("CameraNameRef"=w53, "Display Name"=w46, "ClusterRef"=w54) -> ()  [unwired: 9 in]
  n168 = while {
    tunnel: w56 -> [w319]
    tunnel: w55 -> [_]
    tunnel: [w314] -> _
    tunnel: w47 -> [w310]
    tunnel: w46 -> [w307]
    i -> [w314]
    stop <- FALSE stop-if-true
    n169 = local read "NT Connection"() -> (w311:bool)
    n170 = local read "Rec Mode"() -> (w318:enum32{"Stop", "Record", "Playback"})
    n171 = Bundle("Camera Name Right"="Camera Name Right", w307, "Saved DB Images Info"=w310) -> (w309:T24)  [unwired: 1 in]
    n172 = call <vilib>:"WPI_CameraRead MJPG for Dashboard_2.vi"("Camera Settings"="Camera Settings Right", "Rec Mode"=w318, "NT Connection"=w311, "Capture Info"=w309, "Image in"=w319) -> ("perf info"=w305:cluster{"Bandwidth (Mbps)":dbl, "fps":dbl}, "Active"=w313:bool, "Image\\ out"=w316:T7)  [unwired: 4 in]
    n173 = case shown="False" w313 {
      tunnel: w316 -> [w321 w324]
      tunnel: [w321 w324] -> w312
      tunnel: [_ w323] -> w306
      tunnel: w305 -> [_ w323]
      frame False {
        n174 = Wait Until Next ms Multiple(millisecond multiple=u32 500) -> ()  [unwired: 1 out]
        n175 = property on="Camera Image Right" class="ImageControl"("ROI"=T22 {"Global Rectangle"=[], "Contours"=[]}) -> ()  [unwired: 2 in, 2 out]
      }
      frame True {
      }
    }
    "Camera Image Right" <- w312
    "Right Camera Perf" <- w306
  }
  n176 = register-events(refnum<vi> refnum) -> (reference out=w95:refnum<event-registration>, error out=w94:errorcluster)  [unwired: 2 in]
  n177 = call "Initialize Camera and CheckList.vi"("ListBox in"=w80) -> ()  [unwired: 11 in]
  n178 = call "Adjust Dashboard Window.vi"("Sizing Refnums"=w81, "Size Constraints"=w83, "VI"=w91, "WIn Mode"=w68) -> ()  [unwired: 8 in]
  n179 = call <vilib>:"NT Bind Controls to SmartDashboard.vi"("Bound Control Refs"=w88) -> ()  [unwired: 11 in]
  n180 = vi-ref "Playback Controls.vi"() -> (w96:refnum<vi>)
  n181 = property class="VI"() -> ("Panel"=w98:refnum<vi>)  [unwired: 2 in, 2 out]
  n182 = property class="Pnl"(reference=w98) -> ("Panes[]"=w99:refnum<vi>[])  [unwired: 1 in, 2 out]
  n183 = Index Array(array=w99) -> (element=w97:refnum<vi>)  [unwired: 1 in]
  n184 = control-ref of="Test Tree"() -> (w100:refnum<vi>)
  n185 = while {
    tunnel: [w330] -> _
    tunnel: w100 -> [w329]
    tunnel: w96 -> [w328]
    tunnel: w95 -> [w327]
    tunnel: w94 -> [_]
    tunnel: w91 -> [w326]
    tunnel: w61 -> [w325]
    i -> [w330]
    stop <- FALSE stop-if-true
    n186 = event shown="[0] Timeout" {
      selector: w327 -> [_ _ _ _ _ _ _ _ _ _ _ _ _ _ _ _ _]
      dyn-events: [_ _ _ _ _ _ _ _ _ _ _ _ _ w535 _ _ _] -> _
      timeout: u32 60 ("milliseconds to wait") -> [_ _ _ _ _ _ _ _ _ _ _ _ _ _ _ _ _]
      tunnel: w329 -> [w340 _ _ _ _ _ _ _ _ _ _ _ _ _ _ _ _]
      tunnel: "Test Tree" -> [_ _ _ _ _ _ _ _ w508 w515 w516 w519 w526 _ _ _ _]
      tunnel: w328 -> [_ _ _ _ _ _ _ _ _ _ _ _ _ w537 _ w552 _]
      tunnel: w326 -> [_ _ _ _ _ _ _ _ _ _ _ _ _ w533 _ _ _]
      tunnel: w325 -> [w335 _ _ _ _ _ _ _ _ _ _ _ _ _ _ _ _]
      event Timeout {
        n187 = event-data() -> ()  [unwired: 1 in, 1 out]
        n188 = local read "Mode"() -> (w338:T6)
        n189 = case shown="\"Arm\", Default" "Dashboard Tab" {
          tunnel: w340 -> [_ _ w356 _]
          tunnel: "TestMode/Automatic/" ("Name Pattern") -> [_ _ w355 _]
          tunnel: T25 [{"Operation"=enum."Clear", "Color Box"=14013909}, {"Operation"=enum."Clear", "Color Box"=14013909}, {"Operation"=enum."Clear", "Color Box"=14013909}, {"Operation"=enum."Clear", "Color Box"=14013909}, {"Operation"=enum."Update", "Color Box"=14013909}, {"Operation"=enum."Update", "Color Box"=16777215}, {"Operation"=enum."Clear", "Color Box"=14013909}, {"Operation"=enum."Clear", "Color Box"=14013909}, {"Operation"=enum."Clear", "Color Box"=14013909}] -> [_ _ w348 _]
          tunnel: w338 -> [_ _ w347 _]
          tunnel: u32[] [15790320, 15790320, 15790320, 15790320, 16777215, 16777215, 15790320, 15790320, 15790320] -> [_ _ _ _]
          tunnel: w335 -> [_ w342 _ _]
          frame "Arm", Default {
          }
          frame "Basic" {
            n190 = call <vilib>:"WPI_DashboardUpdateNames.vi"("Controls on Tab"=w342) -> ()  [unwired: 11 in]
          }
          frame "Test" {
            w354 = -2 ("Active Item:Row Number")
            n191 = Index Array(array=w348, index=w347) -> (element=w349:T28)
            n192 = Unbundle(w349) -> ("Operation"=w350:enum16{"Update", "Clear"}, "Color Box"=w351:u32)
            n193 = call <vilib>:"NT Read String.vi"("name"="TestMode/TestName" ("Name")) -> ("value"=w345:string)  [unwired: 8 in, 2 out]
            n194 = call <vilib>:"NT Read and Format Entries as Tree.vi"("Operation"=w350, "Name Pattern"=w355, "Tree Refnum"=w356) -> ()  [unwired: 7 in, 2 out]
            n195 = case shown="\"\"" w345 {
              tunnel: "TestMode/TestProgress" ("Name") -> [w358 _]
              tunnel: "TestMode/TestProgressText" ("Name") -> [w357 _]
              frame Default {
                n196 = call <vilib>:"NT Read Number.vi"("name"=w358) -> ("value"=w359:dbl)  [unwired: 8 in, 2 out]
                n197 = call <vilib>:"NT Read String.vi"("name"=w357) -> ("value"=w360:string)  [unwired: 8 in, 2 out]
                n198 = Bundle("value"=w359, "value"=w360) -> (→"Progress":cluster{"value":dbl, "value":string})  [unwired: 1 in]
              }
              frame "" {
                n199 = property on="Progress" class="Clust (strict)"("Visible"=FALSE) -> ()  [unwired: 2 in, 2 out]
                n200 = local write "Test Name"(u16 0) -> ()
              }
            }
            n201 = property on="Test Tree" class="Tree (strict)"("Active Item Row Number"=w354, "ActiveColNum"=w354, "CellBG"=w351, "Active Item Row Number"=-1 ("Active Item:Row Number"), "CellBG"=u32 5789784 ("Color Box")) -> ()  [unwired: 2 in, 2 out]
          }
          frame "Variables" {
            w366 = string[] ["CameraPublisher", "Usage", "DB"]  # Items to initially close
            n202 = First Call?() -> (First Call?: T/F=w367:bool)
            n203 = control-ref of="Tree"() -> (w368:refnum<vi>)
            n204 = Select(t=w366, s=w367, f=string[] []) -> (s? t:f=w364:string[])
            n205 = call <vilib>:"NT Read and Format Entries as Tree.vi"("Tags to  Close"=w364, "Tree Refnum"=w368) -> ()  [unwired: 8 in, 2 out]
          }
        }
        n206 = call <vilib>:"NT Connection Info.vi"() -> ("Connected"=→"NT Connection":bool)  [unwired: 11 in]
      }
      event "Test Tree": Value Change {
        # "Show appropriate\ncontrols"
        n207 = event-data() -> ("CtlRef"=w372:refnum<vi>, "NewVal"=w370:string)  [unwired: 1 in]
        n208 = call <vilib>:"WPI_UtilitiesGetTreeIOName.vi"("NewVal"=w370, "TreeControl in"=w372) -> ("I/O Name"=w373:string)  [unwired: 9 in]
        n209 = case shown="\"Camera\"" w373 {
          selector: w373 -> [_ w380 _ w402 w411 _]
          tunnel: w370 -> [_ _ w399 w401 _ w418]
          tunnel: cluster{string[]}[] [{["640x480", "320x240", "160x120"]}, {["Auto", "Fixed indoor", "Fixed outdoor 1", "Fixed outdoor 2", "Fixed fluorescent 1", "Fixed fluorescent 2", "Hold current"]}, {["Auto", "Flicker-free 50 Hz", "Flicker-free 60 Hz", "Hold current"]}, {["None", "Prioritize frame rate", "Prioritize image quality"]}, {["Monochrome", "Color"]}] -> [_ _ _ _ _ w417]
          frame Default {
            w375 = FALSE ("Visible")
            w374 = FALSE ("Visible")
            n210 = property on="Motor" class="Clust (strict)"("Visible"=w374) -> ()  [unwired: 2 in, 2 out]
            n211 = property on="Test Ring" class="Ring (strict)"("Visible"=w374) -> ()  [unwired: 2 in, 2 out]
            n212 = property on="Rev/Fwd" class="Clust (strict)"("Visible"=w375) -> ()  [unwired: 2 in, 2 out]
            n213 = property on="On/Off" class="Bool (strict)"("Visible"=w375) -> ()  [unwired: 2 in, 2 out]
            n214 = property on="Test Slider" class="Slide (strict)"("Visible"=w375) -> ()  [unwired: 2 in, 2 out]
          }
          frame "Analog Out", "Motor", "PWM" {
            w381 = FALSE ("Visible")
            n215 = case shown="\"Analog Out\"" w380 {
              tunnel: [1.0 ("Value") -1.0 ("Value") 0.0 ("Value")] -> w379
              tunnel: [255.0 ("Value") 1.0 ("Value") 5.0 ("Value")] -> w378
              tunnel: [128.0 ("Value") 0.0 ("Value") 0.0 ("Value")] -> w377
              tunnel: [64.0 ("Value") 0.5 ("Value") 1.0 ("Value")] -> w376
              frame "PWM" {
              }
              frame "Motor", Default {
              }
              frame "Analog Out" {
              }
            }
            n216 = property on="Motor" class="Clust (strict)"("Visible"=TRUE) -> ()  [unwired: 2 in, 2 out]
            n217 = property on="Value" class="Slide (strict)"("Value"=w377, "Scale.Minimum"=w379, "Scale.Maximum"=w378, "Scale.Increment"=w376) -> ()  [unwired: 2 in, 2 out]
            n218 = property on="On/Off" class="Bool (strict)"("Visible"=w381) -> ()  [unwired: 2 in, 2 out]
            n219 = property on="Test Slider" class="Slide (strict)"("Visible"=w381) -> ()  [unwired: 2 in, 2 out]
            n220 = property on="Test Ring" class="Ring (strict)"("Visible"=w381) -> ()  [unwired: 2 in, 2 out]
            n221 = property on="Rev/Fwd" class="Clust (strict)"("Visible"=w381) -> ()  [unwired: 2 in, 2 out]
          }
          frame "Servo" {
            w397 = FALSE ("Visible")
            n222 = call <vilib>:"NT Read Number.vi"("name"=w399) -> ("value"=w398:dbl)  [unwired: 8 in, 2 out]
            n223 = property on="Test Slider" class="Slide (strict)"("Visible"=TRUE, "Scale.Maximum"=170.0 ("Scale.Range:Maximum")) -> ()  [unwired: 2 in, 2 out]
            n224 = local write "Test Slider"(w398) -> ()
            n225 = property on="Motor" class="Clust (strict)"("Visible"=w397) -> ()  [unwired: 2 in, 2 out]
            n226 = property on="Rev/Fwd" class="Clust (strict)"("Visible"=w397) -> ()  [unwired: 2 in, 2 out]
            n227 = property on="On/Off" class="Bool (strict)"("Visible"=w397) -> ()  [unwired: 2 in, 2 out]
            n228 = property on="Test Ring" class="Ring (strict)"("Visible"=w397) -> ()  [unwired: 2 in, 2 out]
          }
          frame "Relay", "Solenoid" {
            w400 = FALSE ("Visible")
            n229 = property on="Motor" class="Clust (strict)"("Visible"=w400) -> ()  [unwired: 2 in, 2 out]
            n230 = property on="Test Slider" class="Slide (strict)"("Visible"=w400) -> ()  [unwired: 2 in, 2 out]
            n231 = Search and Replace String(input string=w401, search string="/Value  **", replace string="/Direction") -> (result string=w407:string)  [unwired: 5 in, 3 out]
            n232 = property on="Test Ring" class="Ring (strict)"("Visible"=w400) -> ()  [unwired: 2 in, 2 out]
            n233 = call <vilib>:"NT Read String.vi"("name"=w407) -> ("value"=w405:string)  [unwired: 8 in, 2 out]
            n234 = Equal?(x="Both directions", y=w405) -> (x = y?=w403:bool)
            n235 = Not(x=w403) -> (.not. x?=w404:bool)
            n236 = property on="Rev/Fwd" class="Clust (strict)"("Visible"=w403) -> ()  [unwired: 2 in, 2 out]
            n237 = property on="On/Off" class="Bool (strict)"("Visible"=w404, "Caption.Text"=w402) -> ()  [unwired: 2 in, 2 out]
          }
          frame "Compressor", "Digital Out" {
            w410 = FALSE ("Visible")
            # "Get direction and finish"
            n238 = property on="Motor" class="Clust (strict)"("Visible"=w410) -> ()  [unwired: 2 in, 2 out]
            n239 = property on="Test Slider" class="Slide (strict)"("Visible"=w410) -> ()  [unwired: 2 in, 2 out]
            n240 = property on="Test Ring" class="Ring (strict)"("Visible"=w410) -> ()  [unwired: 2 in, 2 out]
            n241 = property on="On/Off" class="Bool (strict)"("Visible"=TRUE, "Caption.Text"=w411) -> ()  [unwired: 2 in, 2 out]
            n242 = property on="Rev/Fwd" class="Clust (strict)"("Visible"=FALSE) -> ()  [unwired: 2 in, 2 out]
          }
          frame "Camera" {
            n243 = call <vilib>:"NT_Get Last Path Segment.vi"("String in"=w418) -> ("String out"=w419:string)  [unwired: 10 in]
            n244 = property on="On/Off" class="Bool (strict)"("Visible"=FALSE) -> ()  [unwired: 2 in, 2 out]
            n245 = property on="Motor" class="Clust (strict)"("Visible"=FALSE) -> ()  [unwired: 2 in, 2 out]
            n246 = property on="Rev/Fwd" class="Clust (strict)"("Visible"=FALSE) -> ()  [unwired: 2 in, 2 out]
            n247 = case shown="\"White Balance  **\"" w419 {
              tunnel: w418 -> [w425 w434 w443 w452 w461 _ w467]
              tunnel: w417 -> [w423 w431 w440 w449 w458 _ _]
              frame "Size  **" {
                n248 = Index Array(array=w423) -> (element=w422:cluster{string[]})  [unwired: 1 in]
                n249 = call <vilib>:"NT Read String.vi"("name"=w425) -> ("value"=w424:string)  [unwired: 8 in, 2 out]
                n250 = Unbundle(w422) -> (w420:string[])
                n251 = Match First String(2:w420, 3:w424) -> (0:w421:i32)  [unwired: 1 out]
                n252 = property on="Test Ring" class="Ring (strict)"("Value"=w421, "Strings []"=w420) -> ()  [unwired: 2 in, 2 out]
                n253 = property on="Test Ring" class="Ring (strict)"("Visible"=TRUE) -> ()  [unwired: 2 in, 2 out]
                n254 = property on="Test Slider" class="Slide (strict)"("Visible"=FALSE) -> ()  [unwired: 2 in, 2 out]
              }
              frame "White Balance  **" {
                n255 = Index Array(array=w431, index=1) -> (element=w432:cluster{string[]})
                n256 = call <vilib>:"NT Read String.vi"("name"=w434) -> ("value"=w433:string)  [unwired: 8 in, 2 out]
                n257 = Unbundle(w432) -> (w429:string[])
                n258 = Match First String(2:w429, 3:w433) -> (0:w428:i32)  [unwired: 1 out]
                n259 = property on="Test Ring" class="Ring (strict)"("Value"=w428, "Strings []"=w429) -> ()  [unwired: 2 in, 2 out]
                n260 = property on="Test Ring" class="Ring (strict)"("Visible"=TRUE) -> ()  [unwired: 2 in, 2 out]
                n261 = property on="Test Slider" class="Slide (strict)"("Visible"=FALSE) -> ()  [unwired: 2 in, 2 out]
              }
              frame "Exposure  **" {
                n262 = Index Array(array=w440, index=2) -> (element=w441:cluster{string[]})
                n263 = call <vilib>:"NT Read String.vi"("name"=w443) -> ("value"=w442:string)  [unwired: 8 in, 2 out]
                n264 = Unbundle(w441) -> (w437:string[])
                n265 = Match First String(2:w437, 3:w442) -> (0:w438:i32)  [unwired: 1 out]
                n266 = property on="Test Ring" class="Ring (strict)"("Value"=w438, "Strings []"=w437) -> ()  [unwired: 2 in, 2 out]
                n267 = property on="Test Ring" class="Ring (strict)"("Visible"=TRUE) -> ()  [unwired: 2 in, 2 out]
                n268 = property on="Test Slider" class="Slide (strict)"("Visible"=FALSE) -> ()  [unwired: 2 in, 2 out]
              }
              frame "Exposure Priority  **" {
                n269 = Index Array(array=w449, index=3) -> (element=w450:cluster{string[]})
                n270 = call <vilib>:"NT Read String.vi"("name"=w452) -> ("value"=w451:string)  [unwired: 8 in, 2 out]
                n271 = Unbundle(w450) -> (w446:string[])
                n272 = Match First String(2:w446, 3:w451) -> (0:w447:i32)  [unwired: 1 out]
                n273 = property on="Test Ring" class="Ring (strict)"("Value"=w447, "Strings []"=w446) -> ()  [unwired: 2 in, 2 out]
                n274 = property on="Test Ring" class="Ring (strict)"("Visible"=TRUE) -> ()  [unwired: 2 in, 2 out]
                n275 = property on="Test Slider" class="Slide (strict)"("Visible"=FALSE) -> ()  [unwired: 2 in, 2 out]
              }
              frame "Color Enable  **" {
                n276 = Index Array(array=w458, index=4) -> (element=w459:cluster{string[]})
                n277 = call <vilib>:"NT Read String.vi"("name"=w461) -> ("value"=w460:string)  [unwired: 8 in, 2 out]
                n278 = Unbundle(w459) -> (w455:string[])
                n279 = Match First String(2:w455, 3:w460) -> (0:w456:i32)  [unwired: 1 out]
                n280 = property on="Test Ring" class="Ring (strict)"("Value"=w456, "Strings []"=w455) -> ()  [unwired: 2 in, 2 out]
                n281 = property on="Test Ring" class="Ring (strict)"("Visible"=TRUE) -> ()  [unwired: 2 in, 2 out]
                n282 = property on="Test Slider" class="Slide (strict)"("Visible"=FALSE) -> ()  [unwired: 2 in, 2 out]
              }
              frame Default {
                n283 = property on="Test Ring" class="Ring (strict)"("Visible"=FALSE) -> ()  [unwired: 2 in, 2 out]
                n284 = property on="Test Slider" class="Slide (strict)"("Visible"=FALSE) -> ()  [unwired: 2 in, 2 out]
              }
              frame "Brightness  **", "Color Level  **", "Compression  **", "FPS  **", "Sharpness  **" {
                n285 = call <vilib>:"NT Read Number.vi"("name"=w467) -> ("value"=w466:dbl)  [unwired: 8 in, 2 out]
                n286 = local write "Test Slider"(w466) -> ()
                n287 = property on="Test Ring" class="Ring (strict)"("Visible"=FALSE) -> ()  [unwired: 2 in, 2 out]
                n288 = property on="Test Slider" class="Slide (strict)"("Visible"=TRUE, "Scale.Maximum"=100.0 ("Scale.Range:Maximum")) -> ()  [unwired: 2 in, 2 out]
              }
            }
          }
        }
        n289 = property on="Progress" class="Clust (strict)"("Visible"=FALSE) -> ()  [unwired: 2 in, 2 out]
      }
      event "Test Name": Mouse Enter {
        # "Populate the ring with the list of tests"
        n290 = event-data() -> ()  [unwired: 1 in, 1 out]
        n291 = call <vilib>:"NT Read String Array.vi"("name"="TestMode/TestList" ("Name")) -> ("value"=w474:string[])  [unwired: 8 in, 2 out]
        n292 = Build Array (concatenate)("Select the test to run...", w474) -> (w473:string[])
        n293 = property on="Test Name" class="Ring (strict)"("Strings []"=w473) -> ()  [unwired: 2 in, 2 out]
      }
      event "Test Name": Value Change {
        w475 = FALSE ("Visible")
        # "Tell the robot the test name to run"
        n294 = event-data() -> ("NewVal"=w479:u16)  [unwired: 1 in]
        n295 = property on="Test Name" class="Ring (strict)"() -> ("Strings []"=w480:string[])  [unwired: 2 in, 2 out]
        n296 = local write "Progress"(T8 {"Test Progress"=0, "Test Progress Text"=""} ("Progress")) -> ()
        n297 = Index Array(array=w480, index=w479) -> (element=w478:string)
        n298 = call <vilib>:"NT Write String.vi"("value"=w478, "name"="TestMode/TestName" ("Name")) -> ()  [unwired: 9 in, 1 out]
        n299 = property on="Progress" class="Clust (strict)"("Visible"=TRUE) -> ()  [unwired: 2 in, 2 out]
        n300 = property on="Motor" class="Clust (strict)"("Visible"=w475) -> ()  [unwired: 2 in, 2 out]
        n301 = property on="Test Slider" class="Slide (strict)"("Visible"=w475) -> ()  [unwired: 2 in, 2 out]
        n302 = property on="On/Off" class="Bool (strict)"("Visible"=w475) -> ()  [unwired: 2 in, 2 out]
        n303 = property on="Rev/Fwd" class="Clust (strict)"("Visible"=w475) -> ()  [unwired: 2 in, 2 out]
        n304 = property on="Test Ring" class="Ring (strict)"("Visible"=w475) -> ()  [unwired: 2 in, 2 out]
      }
      event "Select Auto": Mouse Enter {
        # "Populate the combo box with the list of autonomous options"
        n305 = event-data() -> ()  [unwired: 1 in, 1 out]
        n306 = call <vilib>:"NT Read String Array.vi"("name"="Auto List" ("Name")) -> ("value"=w482:string[])  [unwired: 8 in, 2 out]
        n307 = property on="Select Auto" class="CmbBox"("Strings[]"=w482) -> ()  [unwired: 2 in, 2 out]
      }
      event "Select Auto": Value Change {
        # "User modified the Auto Selection. Write to NT variable so robot knows."
        n308 = event-data() -> ("NewVal"=w484:string)  [unwired: 1 in]
        n309 = call <vilib>:"NT Write String.vi"("value"=w484, "name"="Auto Selector" ("Name")) -> ()  [unwired: 9 in, 1 out]
      }
      event "CheckList": Double Click {
        # "Shift clears all"
        # "Update symbols on the listbox"
        n310 = event-data() -> ("PlatMods.Shift"=w486:bool, "Row"=w488:i32)  [unwired: 1 in]
        n311 = case shown="True" w486 {
          tunnel: w488 -> [w492 _]
          tunnel: 1 -> [w491 _]
          frame False {
            n312 = property on="CheckList" class="LstBox (strict)"() -> ("Item Symbols"=w490:i32[])  [unwired: 2 in, 2 out]
            n313 = Replace Array Subset(array=w490, new element=w491, index=w492) -> (w489:i32[])
            n314 = property on="CheckList" class="LstBox (strict)"("Item Symbols"=w489) -> ()  [unwired: 2 in, 2 out]
          }
          frame True {
            w493 = 0 ("Top Row")
            n315 = property on="CheckList" class="LstBox (strict)"() -> ("Number of Rows"=w495:u32)  [unwired: 2 in, 2 out]
            n316 = Initialize Array(0, w495) -> (w494:i32[])
            n317 = property on="CheckList" class="LstBox (strict)"("Top Row"=w493, "Value"=w493, "Item Symbols"=w494) -> ()  [unwired: 2 in, 2 out]
          }
        }
      }
      event "CheckList": Key Down {
        # "Update symbols on the listbox\nLeft and right keys check and uncheck"
        n318 = event-data() -> ("VKey"=w498:T26)  [unwired: 1 in]
        n319 = case shown="\"Left\", \"Right\"" w498 {
          selector: w498 -> [w503 _]
          tunnel: eventvkey."Left" ("VKey") -> [w501 _]
          frame "Left", "Right" {
            n320 = Equal?(x=w501, y=w503) -> (x = y?=w502:bool)
            n321 = Select(t=0, s=w502, f=1) -> (s? t:f=w504:i32)
            n322 = property on="CheckList" class="LstBox (strict)"() -> ("Item Symbols"=w507:i32[])  [unwired: 2 in, 2 out]
            n323 = Replace Array Subset(array=w507, new element=w504, index="CheckList") -> (w506:i32[])
            n324 = property on="CheckList" class="LstBox (strict)"("Item Symbols"=w506) -> ()  [unwired: 2 in, 2 out]
          }
          frame Default {
          }
        }
      }
      event "Motor.Enable": Value Change {
        # "When the test mode otor enable helper is set, update that\ntree row item's value"
        n325 = event-data() -> ("NewVal"=w512:bool)  [unwired: 1 in]
        n326 = Unbundle("Motor") -> ("Value"=w511:dbl)  [unwired: 1 out]
        n327 = Select(t=w511, s=w512, f=0.0) -> (s? t:f=w509:dbl)
        n328 = call <vilib>:"NT Write Number.vi"("value"=w509, "name"=w508) -> ()  [unwired: 9 in, 1 out]
      }
      event "Test Slider": Value Change {
        # "When the test mode slider helper is set, update that\ntree row item's value"
        n329 = event-data() -> ("NewVal"=w514:dbl)  [unwired: 1 in]
        n330 = call <vilib>:"NT Write Number.vi"("value"=w514, "name"=w515) -> ()  [unwired: 9 in, 1 out]
      }
      event "On/Off": Value Change {
        # "When the test mode on/off helper value is set, update that\ntree row item's value"
        n331 = event-data() -> ("NewVal"=w518:bool)  [unwired: 1 in]
        n332 = Boolean To (0,1)(Boolean=w518) -> (0, 1=w517:i16)
        n333 = call <vilib>:"NT Write Number.vi"("value"=w517, "name"=w516) -> ()  [unwired: 9 in, 1 out]
      }
      event "Rev/Fwd": Value Change {
        # "When the test mode helper value for relays is set, update that\ntree row item's value"
        n334 = event-data() -> ("NewVal.Forward"=w525:bool, "NewVal.Reverse"=w524:bool)  [unwired: 1 in]
        n335 = Boolean To (0,1)(Boolean=w525) -> (0, 1=w521:i16)
        n336 = Boolean To (0,1)(Boolean=w524) -> (0, 1=w523:i16)
        n337 = Negate(x=w523) -> (-x=w522:i16)
        n338 = Add(x=w521, y=w522) -> (x+y=w520:i16)
        n339 = call <vilib>:"NT Write Number.vi"("value"=w520, "name"=w519) -> ()  [unwired: 9 in, 1 out]
      }
      event "Test Ring": Value Change {
        # "When a test mode helper value is selected from the ring,\nset the tree item's variable to the string value"
        n340 = event-data() -> ("NewVal"=w528:u16)  [unwired: 1 in]
        n341 = property on="Test Ring" class="Ring (strict)"() -> ("Strings []"=w529:string[])  [unwired: 2 in, 2 out]
        n342 = Index Array(array=w529, index=w528) -> (element=w527:string)
        n343 = call <vilib>:"NT Write String.vi"("value"=w527, "name"=w526) -> ()  [unwired: 9 in, 1 out]
      }
      event "Rec Mode": Value Change {
        # "Update globals for recording mode and path to read log from.\nClear when logging and let NetworkTables set path for vision to\nuse."
        n344 = event-data() -> ("NewVal"=w538:enum32{"Stop", "Record", "Playback"})  [unwired: 1 in]
        n345 = global write "WPI_DashboardLogging Global.vi" "Logging Filename"(path "") -> ()
        n346 = global write "WPI_DashboardLogging Global.vi" "Recording"(w538) -> ()
        n347 = case shown="\"Playback\"" w538 {
          tunnel: w537 -> [_ w540 w548]
          tunnel: [_ _ w547] -> w535
          tunnel: [_ _ w546] -> _
          tunnel: w533 -> [_ _ w544]
          tunnel: cluster{i32, i32} {-250, 170} -> [_ _ w543]
          tunnel: [_ _ T27 {"Image Size"=TRUE, "Image Type"=TRUE, "Pixel Value"=TRUE, "ROI Information"=TRUE, "Zoom Factor"=FALSE} ("Image Information Shown:All Elements")] -> w530
          tunnel: [_ _ TRUE ("Zoom Factor")] -> w531
          frame Default {
          }
          frame "Stop", "Record" {
            # "Place Window too"
            n348 = invoke class="VI" method="FP.Close"(reference=w540) -> (reference out=w539:refnum<vi>)  [unwired: 2 in, 2 out]
            n349 = invoke class="VI" method="Abort VI"(reference=w539) -> ()  [unwired: 2 in, 3 out]
          }
          frame "Playback" {
            n350 = call "Open Playback Panel.vi"("Offset"=w543, "DB VI Ref"=w544, "Playback in"=w548) -> ("Playback out"=w545:refnum<vi>)  [unwired: 8 in]
            n351 = register-events(w545) -> (reference out=w547:refnum<event-registration>, error out=w546:errorcluster)  [unwired: 2 in]
          }
        }
        n352 = property on="Camera Image Right" class="ImageControl"("Image Information Shown"=w530, "Image Information Visible"=w531) -> ()  [unwired: 2 in, 2 out]
        n353 = property on="Camera Image" class="ImageControl"("Image Information Shown"=w530, "Image Information Visible"=w531) -> ()  [unwired: 2 in, 2 out]
        n354 = call <vilib>:"WPI_DashboardNT Log FieldName Cache.vi"("Operation"=enum16{"Lookup/Add", "Index", "Clear"}."Clear") -> ()  [unwired: 8 in, 3 out]
      }
      event Panel Close {
        w549 = enum32{"Stop", "Record", "Playback"}."Stop" ("Rec Mode")
        # "Playback window has been closed, abort"
        n355 = event-data() -> ()  [unwired: 1 in, 4 out]
        n356 = local write "Rec Mode"(w549) -> ()
        n357 = global write "WPI_DashboardLogging Global.vi" "Recording"(w549) -> ()
      }
      event Panel Close {
        # "Abort playback window and ourself"
        n358 = event-data() -> ()  [unwired: 1 in, 4 out]
        n359 = invoke class="VI" method="FP.Close"(reference=w552) -> (reference out=w551:refnum<vi>)  [unwired: 2 in, 2 out]
        n360 = invoke class="VI" method="Abort VI"(reference=w551) -> (error out=w550:errorcluster)  [unwired: 2 in, 2 out]
        n361 = invoke class="VI" method="Abort VI"(error in=w550) -> ()  [unwired: 2 in, 3 out]
      }
      event "Tree": Double Click {
        n362 = event-data() -> ("PlatMods"=w558:T29, "Tag"=w555:string)  [unwired: 1 in]
        n363 = Unbundle(w558) -> ("Shift"=w557:bool)  [unwired: 4 out]
        n364 = String Subset(string=w555, length (rest)=1 ("length (rest)")) -> (substring=w554:string)  [unwired: 1 in]
        n365 = Not(x=w557) -> (.not. x?=w556:bool)
        n366 = case shown="\"/\"" w554 {
          tunnel: w555 -> [_ w560]
          tunnel: w556 -> [_ w559]
          frame Default {
          }
          frame "/" {
            n367 = call <vilib>:"NT Update Persistence.vi"("Persistence"=w559, "Name"=w560) -> ()  [unwired: 9 in, 1 out]
          }
        }
      }
    }
  }
  n368 = while {
    tunnel: w97 -> [w562]
    i -> [w565]
    stop <- FALSE stop-if-true
    n369 = Wait (ms)(milliseconds to wait=u32 100) -> ()  [unwired: 1 out]
    n370 = case shown="\"Playback\"" "Rec Mode" {
      tunnel: w565 -> [_ _ w580]
      tunnel: [u32 2829099 ("Base Color") u32 11141120 ("Target Color") w569] -> w561
      frame "Stop", Default {
        # "Reset the color, extra updates don't cost much"
      }
      frame "Record" {
      }
      frame "Playback" {
        # "Playback"
        n371 = Quotient & Remainder(x=w580, y=u32 50 ("milliseconds to wait")) -> (x-y*floor(x/y)=w576:u32)  [unwired: 1 out]
        n372 = Divide(x=w576, y=u32 50 ("milliseconds to wait")) -> (x/y=w573:dbl)
        n373 = Multiply(x=6.283185307179586, y=w573) -> (x*y=w578:dbl)
        n374 = Sine(x=w578) -> (sin(x)=w577:dbl)
        n375 = Absolute Value(x=w577) -> (abs(x)=w570:dbl)
        n376 = call "Interpolate RGB Color.vi"("Proportion"=w570, "Target Color"=u32 30976, "Base Color"=u32 2829099) -> ("Result Color"=w569:u32)  [unwired: 8 in]
      }
    }
    n377 = property class="Pane"(reference=w562, "PaneColor"=w561) -> ()  [unwired: 1 in, 2 out]
  }
  n378 = local write "Dashboard Tab"(T4."Arm" ("Dashboard Tab")) -> ()
  n379 = property on="On/Off" class="Bool (strict)"("Visible"=w69) -> ()  [unwired: 2 in, 2 out]
  n380 = property on="Motor" class="Clust (strict)"("Visible"=w69) -> ()  [unwired: 2 in, 2 out]
  n381 = property on="Progress" class="Clust (strict)"("Visible"=w69) -> ()  [unwired: 2 in, 2 out]
  n382 = property on="Test Ring" class="Ring (strict)"("Visible"=w69) -> ()  [unwired: 2 in, 2 out]
  n383 = property on="Rev/Fwd" class="Clust (strict)"("Visible"=w69) -> ()  [unwired: 2 in, 2 out]
  n384 = while {
    tunnel: u16 1741 ("timeout ms (25000)") -> [w582]
    stop <- FALSE stop-if-true
    n385 = TCP Create Listener(10:w582) -> (0:w581:errorcluster, 3:w583:refnum<k5>)  [unwired: 4 in, 1 out]
    n386 = case shown="No Error" w581 {
      selector: w581 -> [w585 _]
      tunnel: w583 -> [w586 _]
      frame No Error {
        n387 = while {
          tunnel: w586 -> [w589]
          tunnel: w585 -> [w588]
          stop <- FALSE stop-if-true
          n388 = TCP Wait On Listener(8:w588, 11:w589) -> (0:w590:errorcluster, 4:w591:refnum<k5>)  [unwired: 2 in, 3 out]
          n389 = local write "TCP"(w591) -> ()
          n390 = case shown="Error" w590 {
            frame No Error {
            }
            frame Error {
              n391 = Wait (ms)(milliseconds to wait=u32 1000) -> ()  [unwired: 1 out]
            }
          }
        }
      }
      frame Error {
        n392 = Wait (ms)(milliseconds to wait=u32 1000) -> ()  [unwired: 1 out]
      }
    }
  }
  n393 = global write "WPI_DashboardLogging Global.vi" "Recording"(w92) -> ()
  n394 = local write "Rec Mode"(w92) -> ()
  n395 = call <vilib>:"NT Write String.vi"("value"="Select Auto", "name"="Auto Selector" ("Name")) -> ()  [unwired: 9 in, 1 out]
  n396 = control-ref of="Field"() -> (w7:refnum<vi>)
  n397 = property on="Property Node" class="XYGraph (strict)"(reference=w7) -> ("Width"=w9:u32, "Height"=w10:u32)  [unwired: 1 in, 2 out]
  n398 = Divide(x=71.0, y=649.0) -> (x/y=w25:dbl)
  n399 = Divide(x=14.0, y=319.0) -> (x/y=w28:dbl)
  n400 = Multiply(x=w25, y=2.0) -> (x*y=w24:dbl)
  n401 = Multiply(x=w28, y=2.0) -> (x*y=w23:dbl)
  n402 = call "IMAQ Create"("Image Name"="Field image", "Image Type"=w43) -> ("New Image"=w6:T7)  [unwired: 3 in, 1 out]
  n403 = call <vilib>:"Picture to Pixmap.vi"("picture"=w3) -> ("image data"=w5:T30)  [unwired: 9 in, 1 out]
  n404 = Divide(x=67.0, y=319.0) -> (x/y=w18:dbl)
  n405 = Divide(x=12.0, y=649.0) -> (x/y=w17:dbl)
  n406 = Increment(x=w24) -> (x+1=w22:dbl)
  n407 = Increment(x=w23) -> (x+1=w21:dbl)
  n408 = Negate(x=w18) -> (-x=w16:dbl)
  n409 = Increment(x=w18) -> (x+1=w12:dbl)
  n410 = Negate(x=w17) -> (-x=w15:dbl)
  n411 = Increment(x=w17) -> (x+1=w11:dbl)
  n412 = call "Convert LabVIEW Image Data To IMAQ.vi"("Image Data"=w5, "Image In"=w6) -> ("Image Out"=w4:T7)  [unwired: 8 in, 1 out]
  n413 = Multiply(x=w9, y=w22) -> (x*y=w20:dbl)
  n414 = Multiply(x=w10, y=w21) -> (x*y=w19:dbl)
  n415 = Multiply(x=w12, y=w10) -> (x*y=w14:dbl)
  n416 = Multiply(x=w11, y=w9) -> (x*y=w13:dbl)
  n417 = call "IMAQ Resample"("X Resolution"=w20, "Y Resolution"=w19, "Image Src"=w4) -> ("Image Dst Out"=w42:T7)  [unwired: 7 in, 1 out]
  n418 = Multiply(x=w16, y=w14) -> (x*y=w34:dbl)
  n419 = Multiply(x=w15, y=w13) -> (x*y=w35:dbl)
  n420 = call "IMAQ ColorImageToArray"("Image"=w42) -> ("Image Pixels (U32)"=w41:u32[][])  [unwired: 3 in, 2 out]
  n421 = Bundle(cluster=cluster{"x":i16, "y":i16} {"x"=0, "y"=0} ("top left point(0, 0)"), "x"=w34, "y"=w35) -> (w33:cluster{"x":i16, "y":i16})
  n422 = call-poly <vilib>:"Draw Unflattened Pixmap.vi"("top left point(0, 0)"=w33, "data (RGB format)"=w41) -> ("new picture"=w8:picture)  [unwired: 7 in]
  n423 = property class="XYGraph (strict)"(reference=w7, "PlotImages.Back"=w8) -> (reference out=w2:refnum<vi>)  [unwired: 1 in, 1 out]
  n424 = disable-structure shown="Disabled" {
    disable-tunnel: w2 -> [w598 _]
    frame Disabled {
      n425 = property class="XYGraph (strict)"(reference=w598) -> (reference out=w595:refnum<vi>, "CrsrList"=w597:T32)  [unwired: 1 in, 1 out]
      n426 = in-place {
        n427 = in-place-array #7(w597, 0) -> (w600:T33)
        n428 = Bundle By Name(cluster=w600, "Position"=T31 {"X"=8.270875, "Y"=4.105275} ("Cursor.Cursor Position")) -> (w599:T33)
        n429 = in-place-array #7(w599) -> (w596:T32)  [unwired: 1 out]
      }
      n430 = property class="XYGraph (strict)"(reference=w595, "CrsrList"=w596) -> ()  [unwired: 1 in, 2 out]
    }
    frame Enabled {
    }
  }
